vi "B2G2_UiStdControl.vi"() -> ()   [LabVIEW 2011]
panel:
  in  "stop":bool
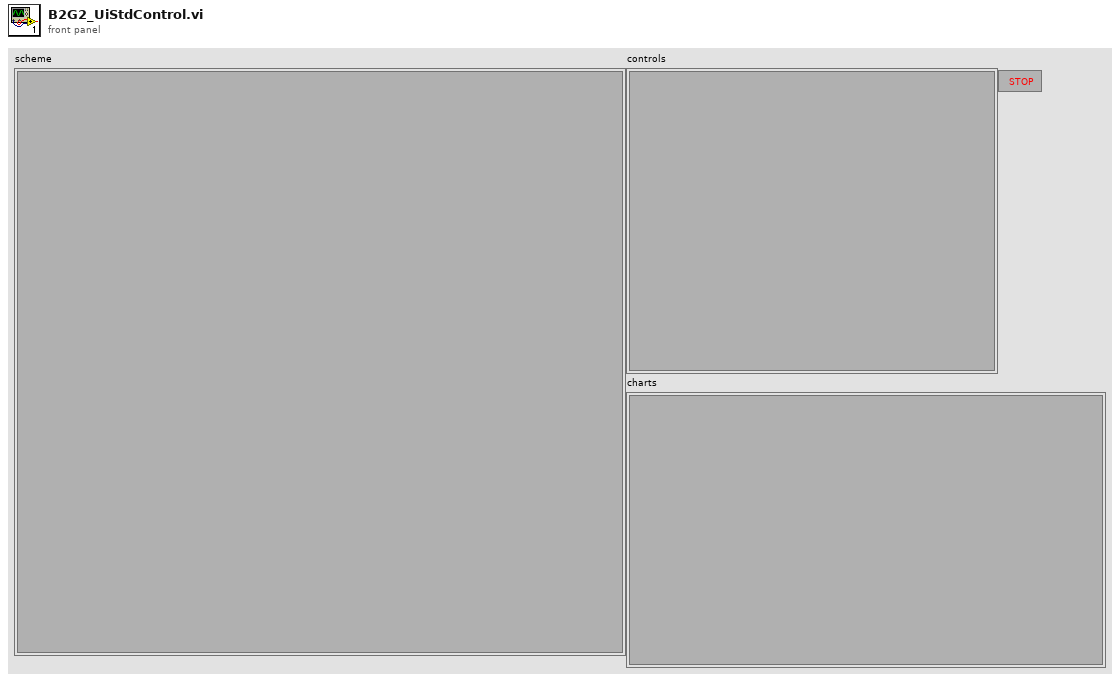
[diagram p1: front panel]
types:
  T1 = enum16{"Always On", "Always Off", "Off While Running"}
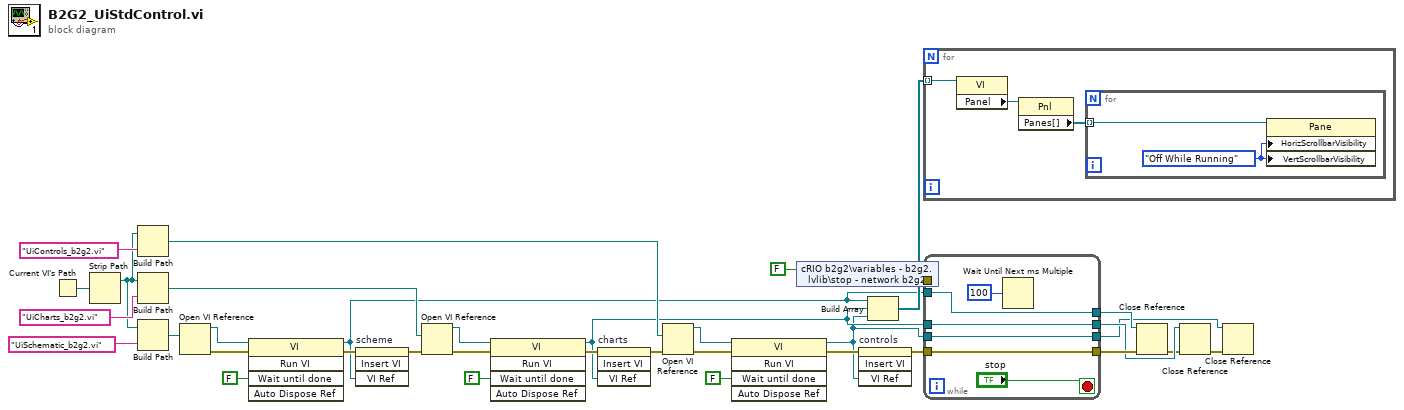
[diagram p0: block diagram]
diagram:
  n1 = Current VI's Path() -> (path=w6:path)
  n2 = Strip Path(path=w6) -> (stripped path=w5:path)  [unwired: 1 out]
  n3 = Build Path(base path=w5, name or relative path="UiControls_b2g2.vi") -> (appended path=w12:path)
  n4 = Build Path(base path=w5, name or relative path="UiCharts_b2g2.vi") -> (appended path=w21:path)
  n5 = Build Path(base path=w5, name or relative path="UiSchematic_b2g2.vi") -> (appended path=w26:path)
  n6 = Open VI Reference(vi path=w26) -> (vi reference=w33:refnum<vi>, error out=w32:errorcluster)  [unwired: 5 in]
  n7 = invoke class="VI" method="Run VI"(reference=w33, error in=w32, "Wait until done"=FALSE) -> (reference out=w3:refnum<vi>, error out=w29:errorcluster)  [unwired: 2 in, 3 out]
  n8 = invoke on="scheme" class="SubPanel" method="Insert VI"(error in=w29, "VI Ref"=w3) -> (error out=w18:errorcluster)  [unwired: 2 in, 3 out]
  n9 = Open VI Reference(vi path=w21, error in (no error)=w18) -> (vi reference=w25:refnum<vi>, error out=w24:errorcluster)  [unwired: 4 in]
  n10 = invoke class="VI" method="Run VI"(reference=w25, error in=w24, "Wait until done"=FALSE) -> (reference out=w2:refnum<vi>, error out=w20:errorcluster)  [unwired: 2 in, 3 out]
  n11 = invoke on="charts" class="SubPanel" method="Insert VI"(error in=w20, "VI Ref"=w2) -> (error out=w10:errorcluster)  [unwired: 2 in, 3 out]
  n12 = Open VI Reference(vi path=w12, error in (no error)=w10) -> (vi reference=w16:refnum<vi>, error out=w15:errorcluster)  [unwired: 4 in]
  n13 = invoke class="VI" method="Run VI"(reference=w16, error in=w15, "Wait until done"=FALSE) -> (reference out=w1:refnum<vi>, error out=w11:errorcluster)  [unwired: 2 in, 3 out]
  n14 = shared-variable "cRIO b2g2\\variables - b2g2.lvlib\\stop - network b2g2"(FALSE ("stop - network")) -> (error out=w35:errorcluster)  [unwired: 1 in]
  n15 = invoke on="controls" class="SubPanel" method="Insert VI"(error in=w11, "VI Ref"=w1) -> (error out=w9:errorcluster)  [unwired: 2 in, 3 out]
  n16 = Build Array(w3, w2, w1) -> (w4:refnum<vi>[])
  n17 = for {
    tunnel: w4 -> [w37] mode=indexing
    n18 = property class="VI"(reference=w37) -> ("Panel"=w36:refnum<vi>)  [unwired: 1 in, 2 out]
    n19 = property class="Pnl"(reference=w36) -> ("Panes[]"=w38:refnum<vi>[])  [unwired: 1 in, 2 out]
    n20 = for {
      tunnel: w38 -> [w40] mode=indexing
      w39 = T1."Off While Running" ("Scrollbar Visibility")
      n21 = property class="Pane"(reference=w40, "HorizScrollbarVisibility"=w39, "VertScrollbarVisibility"=w39) -> ()  [unwired: 1 in, 2 out]
    }
  }
  n22 = while {
    tunnel: w35 -> [_]
    tunnel: [w44] -> w28
    tunnel: w3 -> [w44]
    tunnel: [w43] -> w27
    tunnel: w9 -> [w43]
    tunnel: w2 -> [w42]
    tunnel: [w42] -> w19
    tunnel: [w41] -> w7
    tunnel: w1 -> [w41]
    stop <- "stop" stop-if-true
    n23 = Wait Until Next ms Multiple(millisecond multiple=u32 100) -> ()  [unwired: 1 out]
  }
  n24 = Close Reference(reference=w28, error in (no error)=w27) -> (error out=w17:errorcluster)
  n25 = Close Reference(reference=w19, error in (no error)=w17) -> (error out=w8:errorcluster)
  n26 = Close Reference(reference=w7, error in (no error)=w8) -> ()  [unwired: 1 out]
